vi "Get Register Map.vi"(6 "offset":i32, 8 "error in (no error)":errorcluster, 11 "bitfile xml in":string) -> (0 "error out":errorcluster, 2 "register map":T1[](array[typedef]) {"Address" format="%.0x"}, 4 "offset past EndTag":i32)   [LabVIEW 2010, in "FPGA Bitfile Utility.lvlib"]
uses:
  <userlib>/_FPGA Interface Advanced Tools/FPGA Bitfile Utility/FPGA Bitfile Utility.lvlib
  <vilib>/rvi/Bitfile/nirviControlStructure.ctl
  <vilib>/rvi/Bitfile/nirviTypdefDescription.ctl
  <vilib>/rvi/Bitfile/nirviMechanicalAction.ctl
  <vilib>/rvi/Bitfile/nirviSubControlStructure.ctl
  <vilib>/rvi/Bitfile/nirviClusterElementControl.ctl
  <vilib>/rvi/Utilities/XML/nirviXML_GetValue_String.vi
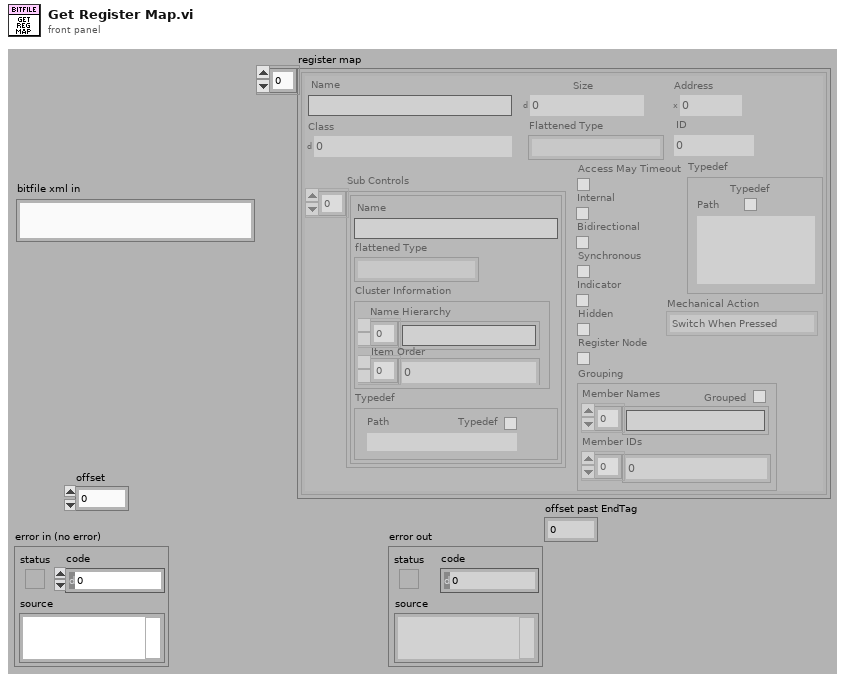
[diagram p1: front panel]
types:
  T1 = typedef "nirviControlStructure.ctl" = cluster{"Name":string, "Hidden":bool, "Indicator":bool, "Flattened Type":string, "Grouping":cluster{"Grouped":bool, "Member Names":string[], "Member IDs":u32[]}, "Address":u32, "Size":u32, "Class":u32, "Internal":bool, "Typedef":T2, "ID":u32, "Bidirectional":bool, "Synchronous":bool, "Mechanical Action":T3, "Sub Controls":T4[], "Access May Timeout":bool, "Register Node":bool}
  T2 = typedef "nirviTypdefDescription.ctl" = cluster{"Typedef":bool, "Path":path}
  T3 = typedef "nirviMechanicalAction.ctl" = enum8{"Switch When Pressed", "Switch When Released", "Switch Until Released", "Latch When Pressed", "Latch When Released", "Latch Until Released"}
  T4 = typedef "nirviSubControlStructure.ctl" = cluster{"Name":string, "flattened Type":string, "Cluster Information":T5, "Typedef":T2}
  T5 = typedef "nirviClusterElementControl.ctl" = cluster{"Name Hierarchy":string[], "Item Order":u32[]}
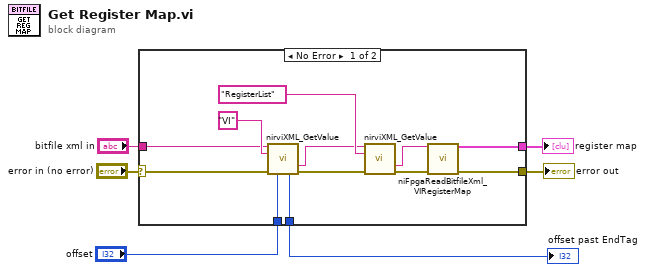
[diagram p0: block diagram]
diagram:
  n1 = case shown="No Error" "error in (no error)" {
    selector: "error in (no error)" -> [w12 w20]
    tunnel: [w11 w20] -> w5
    tunnel: [w10 _] -> w4
    tunnel: "bitfile xml in" -> [w9 _]
    tunnel: "offset" -> [w8 w19]
    tunnel: [w7 w19] -> w1
    frame No Error {
      n2 = call-poly <vilib>:"nirviXML_GetValue.vi"("xml string in"=w9, "tag name in"="VI" ("tag"), "error in (no error)"=w12, "offset"=w8) -> ("value"=w17:string, "offset past EndTag"=w7:i32, "error out"=w14:errorcluster)  [unwired: 1 in, 8 out]
      n3 = call-poly <vilib>:"nirviXML_GetValue.vi"("xml string in"=w17, "tag name in"="RegisterList" ("tag"), "error in (no error)"=w14) -> ("value"=w15:string, "error out"=w13:errorcluster)  [unwired: 2 in, 9 out]
      n4 = call <vilib>:"niFpgaReadBitfileXml_VIRegisterMap.vi"("register map xml"=w15, "error in (no error)"=w13) -> ("register map"=w10:T1[], "error out"=w11:errorcluster)  [unwired: 12 out]
    }
    frame Error {
    }
  }
  "error out" <- w5
  "register map" <- w4
  "offset past EndTag" <- w1
